vi "Read PNG File Metadata.vi"(8 "Error In":errorcluster, 11 "File Path":path) -> (0 "Error Out":errorcluster, 1 "PNG Metadata":T1, 3 "Metadata Text Fields":string[](array[string]))   [LabVIEW 2021, in "Files.lvlib"]
uses:
  Files/Files.lvlib
  Files/PNG/PNG Metadata.ctl
  Files/PNG/PNG Header.ctl
  Files/PNG/PNG Pixel Dimension.ctl
  Files/PNG/PNG Time Last Modified.ctl
  <vilib>/Utility/error.llb/Error Cluster From Error Code.vi
  <vilib>/ErrorRing/Error Ring.xnode
panel:
  out "Fields":string[](array[string])
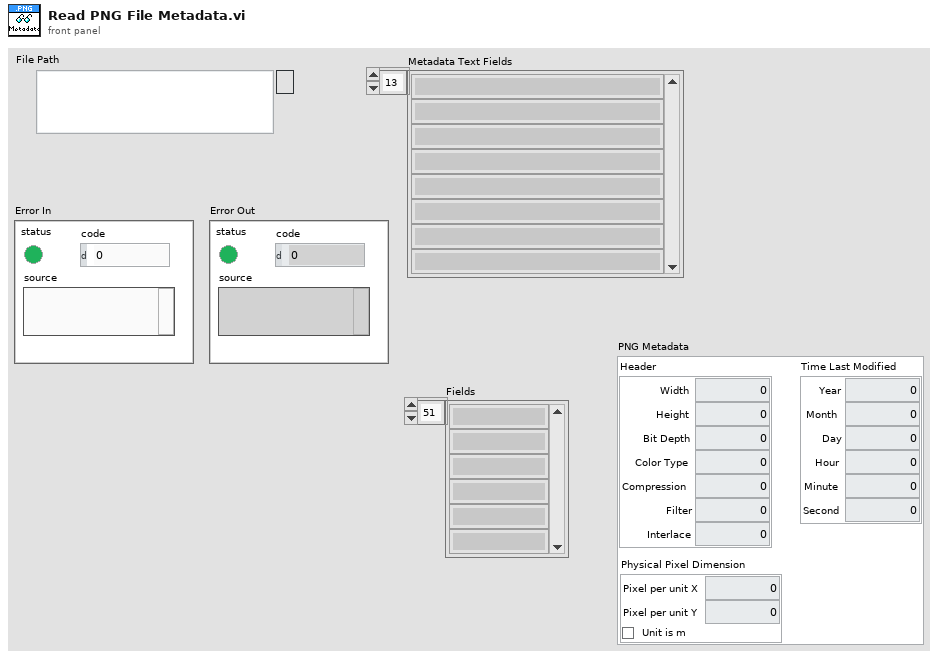
[diagram p1: front panel]
types:
  T1 = typedef "Files.lvlib/PNG Metadata.ctl" = cluster{"Header":T2, "Physical Pixel Dimension":T3, "Time Last Modified":T4}
  T2 = typedef "Files.lvlib/PNG Header.ctl" = cluster{"Width":u32, "Height":u32, "Bit Depth":u8, "Color Type":u8, "Compression":u8, "Filter":u8, "Interlace":u8}
  T3 = typedef "Files.lvlib/PNG Pixel Dimension.ctl" = cluster{"Pixel per unit X":u32, "Pixel per unit Y":u32, "Unit is m":bool}
  T4 = typedef "Files.lvlib/PNG Time Last Modified.ctl" = cluster{"Year":u16, "Month":u8, "Day":u8, "Hour":u8, "Minute":u8, "Second":u8}
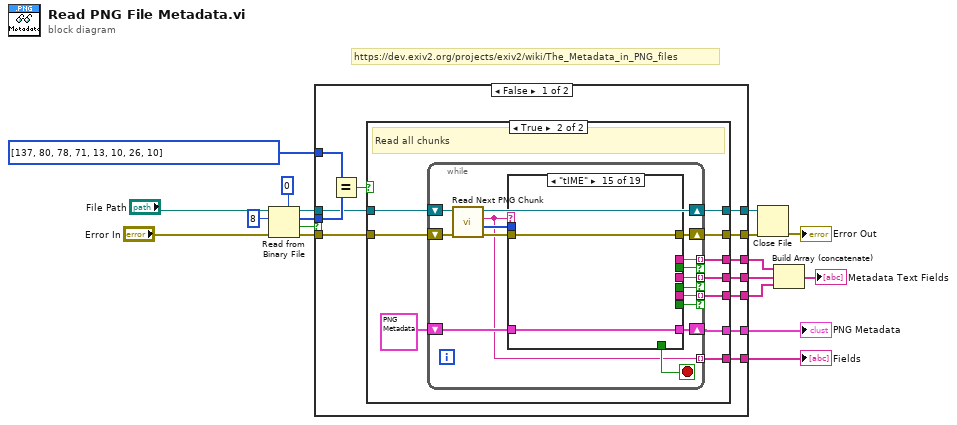
[diagram p0: block diagram]
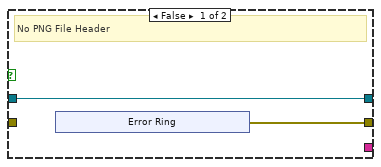
[diagram p2: hidden frame]
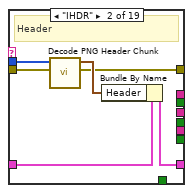
[diagram p4: hidden frame]
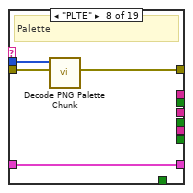
[diagram p10: hidden frame]
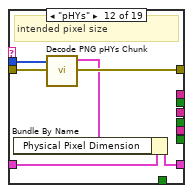
[diagram p14: hidden frame]
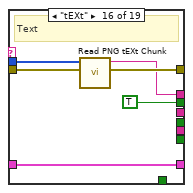
[diagram p17: hidden frame]
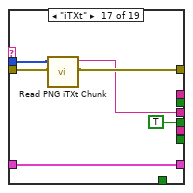
[diagram p18: hidden frame]
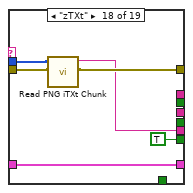
[diagram p19: hidden frame]
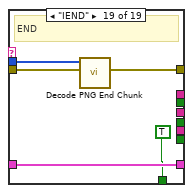
[diagram p20: hidden frame]
diagram:
  # "https://dev.exiv2.org/projects/exiv2/wiki/The_Metadata_in_PNG_files"
  n1 = Read from Binary File(5:u8 0, 8:"Error In", 10:8 ("count (1)"), 11:"File Path") -> (0:w10:errorcluster, 1:w12:bool, 2:w13:u8[], 3:w9:refnum<file>)  [unwired: 2 in]
  n2 = case shown="False" w12 {
    tunnel: w13 -> [w30 _]
    tunnel: u8[] [137, 80, 78, 71, 13, 10, 26, 10] ("data") -> [w29 _]
    tunnel: w10 -> [w25 w127]
    tunnel: w9 -> [w27 w126]
    tunnel: [w26 w126] -> w8
    tunnel: [w24 w127] -> w7
    tunnel: [w23 _] -> w6
    tunnel: [w22 _] -> w5
    tunnel: [w21 _] -> w4
    tunnel: [w20 _] -> w2
    tunnel: [w19 _] -> w1
    frame False {
      n3 = Equal?(x=w29, y=w30) -> (x = y?=w28:bool)
      n4 = case shown="True" w28 {
        tunnel: w27 -> [w32 w46]
        tunnel: [w32 w45] -> w26
        tunnel: w25 -> [_ w44]
        tunnel: [w31 w43] -> w24
        tunnel: [_ w41] -> w23
        tunnel: [_ w40] -> w22
        tunnel: [_ w39] -> w21
        tunnel: [_ w38] -> w20
        tunnel: [_ w37] -> w19
        frame False {
          # "No PNG File Header"
          n5 = xnode "Error Ring"() -> ("error out"=w31:errorcluster)
        }
        frame True {
          # "Read all chunks"
          n6 = while {
            shift-right: [w61] -> w45
            shift-left: w46 -> [w62]
            shift-right: [w57] -> w43
            shift-left: w44 -> [w60]
            shift-right: [w55] -> w41
            shift-left: T1 {"Header"={"Width"=0, "Height"=0, "Bit Depth"=0, "Color Type"=0, "Compression"=0, "Filter"=0, "Interlace"=0}, "Physical Pixel Dimension"={"Pixel per unit X"=0, "Pixel per unit Y"=0, "Unit is m"=FALSE}, "Time Last Modified"={"Year"=0, "Month"=0, "Day"=0, "Hour"=0, "Minute"=0, "Second"=0}} ("PNG Metadata") -> [w56]
            tunnel: [w53] -> w40 mode=indexing if=w52
            tunnel: [w51] -> w39 mode=indexing
            tunnel: [w50] -> w38 mode=indexing if=w49
            tunnel: [w48] -> w37 mode=indexing if=w47
            stop <- w54 stop-if-true
            n7 = call "Read Next PNG Chunk.vi"("error in (no error)"=w60, "Byte Stream File in"=w62) -> ("error out"=w58:errorcluster, "data"=w59:u8[], "Type"=w51:string, "Byte Stream File out"=w61:refnum<file>)  [unwired: 4 in, 2 out]
            n8 = case shown="\"tIME\"" w51 {
              tunnel: w59 -> [_ w70 _ _ _ _ _ w84 _ _ _ w95 _ _ _ w105 w113 w119 w122]
              tunnel: w58 -> [w64 w66 w72 w74 w76 w78 w80 w83 w86 w88 w90 w94 w98 w100 w101 w108 w112 w118 w125]
              tunnel: [w64 w65 w72 w74 w76 w78 w80 w82 w86 w88 w90 w93 w98 w100 w101 w106 w111 w117 w123] -> w57
              tunnel: w56 -> [w63 w69 w71 w73 w75 w77 w79 w81 w85 w87 w89 w96 w97 w99 w102 w107 w114 w120 w124]
              tunnel: [w63 w68 w71 w73 w75 w77 w79 w81 w85 w87 w89 w92 w97 w99 w102 w107 w114 w120 w124] -> w55
              tunnel: [_ _ _ _ _ _ _ _ _ _ _ _ _ _ _ _ _ _ TRUE] -> w54
              tunnel: [_ _ _ _ _ _ _ _ _ _ _ _ _ _ _ w104 _ _ _] -> w53
              tunnel: [_ _ _ _ _ _ _ _ _ _ _ _ _ _ _ TRUE _ _ _] -> w52
              tunnel: [_ _ _ _ _ _ _ _ _ _ _ _ _ _ _ _ w110 _ _] -> w50
              tunnel: [_ _ _ _ _ _ _ _ _ _ _ _ _ _ _ _ TRUE _ _] -> w49
              tunnel: [_ _ _ _ _ _ _ _ _ _ _ _ _ _ _ _ _ w116 _] -> w48
              tunnel: [_ _ _ _ _ _ _ _ _ _ _ _ _ _ _ _ _ TRUE _] -> w47
              frame "", Default {
              }
              frame "IHDR" {
                # "Header"
                n9 = call "Decode PNG Header Chunk.vi"("error in (no error)"=w66, "data"=w70) -> ("error out"=w65:errorcluster, "Header"=w67:T2)  [unwired: 8 in]
                n10 = Bundle By Name(cluster=w69, "Header"=w67) -> (w68:T1)
              }
              frame "cHRM" {
                # "chromaticiy"
              }
              frame "gAMA" {
                # "gamma values"
              }
              frame "iCCP" {
                # "ICC color profile"
              }
              frame "sBIT" {
                # "color-accuracy"
              }
              frame "sRGB" {
                # "standard sRGB color space"
              }
              frame "PLTE" {
                # "Palette"
                n11 = call "Decode PNG Palette Chunk.vi"("error in (no error)"=w83, "data"=w84) -> ("error out"=w82:errorcluster)  [unwired: 8 in, 1 out]
              }
              frame "bKGD" {
                # "default background color"
              }
              frame "hIST" {
                # "histogram"
              }
              frame "tRNS" {
                # "transparency information"
              }
              frame "pHYs" {
                # "intended pixel size"
                n12 = call "Decode PNG pHYs Chunk.vi"("error in (no error)"=w94, "data"=w95) -> ("error out"=w93:errorcluster, "Pixel Dimension"=w91:T3)  [unwired: 8 in]
                n13 = Bundle By Name(cluster=w96, "Physical Pixel Dimension"=w91) -> (w92:T1)
              }
              frame "sPLT" {
                # "palette if all colors unavailable"
              }
              frame "IDAT" {
                # "data"
              }
              frame "tIME" {
              }
              frame "tEXt" {
                # "Text"
                n14 = call "Read PNG tEXt Chunk.vi"("error in (no error)"=w108, "data"=w105) -> ("error out"=w106:errorcluster, "String"=w104:string)  [unwired: 8 in]
              }
              frame "iTXt" {
                n15 = call "Read PNG iTXt Chunk.vi"("error in (no error)"=w112, "data"=w113) -> ("error out"=w111:errorcluster, "String"=w110:string)  [unwired: 8 in]
              }
              frame "zTXt" {
                n16 = call "Read PNG iTXt Chunk.vi"("error in (no error)"=w118, "data"=w119) -> ("error out"=w117:errorcluster, "String"=w116:string)  [unwired: 8 in]
              }
              frame "IEND" {
                # "END"
                n17 = call "Decode PNG End Chunk.vi"("error in (no error)"=w125, "data"=w122) -> ("error out"=w123:errorcluster)  [unwired: 8 in, 1 out]
              }
            }
          }
        }
      }
    }
    frame True {
      # "cancelled"
    }
  }
  "PNG Metadata" <- w6
  "Fields" <- w4
  n18 = Close File(refnum=w8, error in=w7) -> (error out=→"Error Out":errorcluster)  [unwired: 1 out]
  n19 = Build Array (concatenate)(w5, w2, w1) -> (→"Metadata Text Fields":string[])
